vi "Get Icon From File.vi"(8 "错误输入（无错误）":errorcluster, 11 "Path":path) -> (0 "错误输出":errorcluster, 3 "Get Shell Icon Of File":T1)   [LabVIEW 2012, in "Application.lvlib"]
uses:
  Application.lvlib
  <vilib>/picture/picture.llb/imagedata.ctl
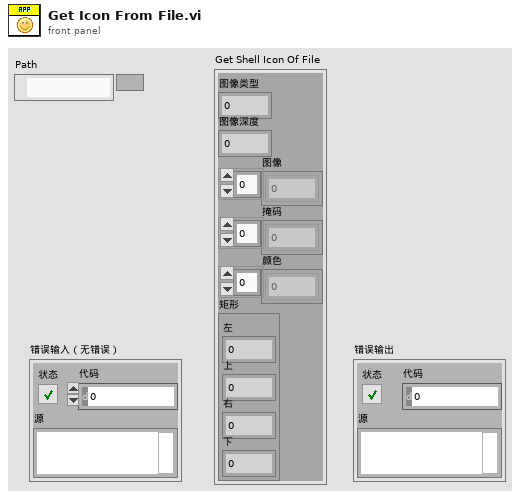
[diagram p1: front panel]
types:
  T1 = typedef "imagedata.ctl" = cluster{"image type":i32, "image depth":i32, "image":u8[], "mask":u8[], "colors":u32[], "Rectangle":cluster{"left":i16, "top":i16, "right":i16, "bottom":i16}}
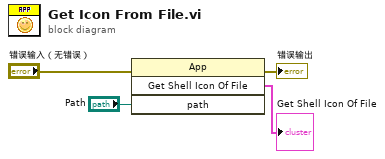
[diagram p0: block diagram]
diagram:
  n1 = invoke class="App" method="Get Shell Icon Of File"(error in="错误输入（无错误）", "path"="Path") -> (error out=→"错误输出":errorcluster, "GetShellIconOfFile"=→"Get Shell Icon Of File":T1)  [unwired: 2 in, 2 out]
